vi "Initialize State.vi"(7 "dialog VI refnum":refnum<vi>, 8 "error in":errorcluster, 10 "VI refs":refnum<vi>[](array[refnum]), 11 "tree refnum":refnum<vi>) -> (0 "error out":errorcluster, 3 "state out":T1)   [LabVIEW 2010, in "NI_SE_Config Front Panel Layout.lvlib"]
uses:
  NI_SE_Config Front Panel Layout.lvlib
  State.ctl
  VI Info.ctl
  VI Panel Layout/VI Panel Layout.lvclass
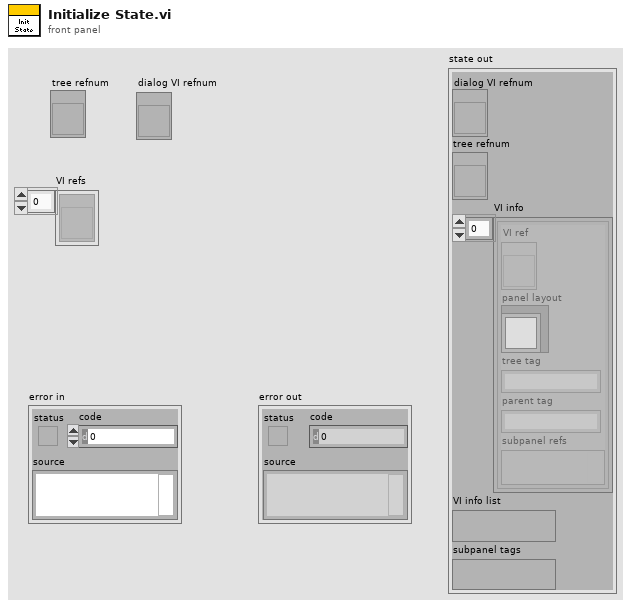
[diagram p1: front panel]
types:
  T1 = typedef "NI_SE_Config Front Panel Layout.lvlib/State.ctl" = cluster{"dialog VI refnum":refnum<vi>, "tree refnum":refnum<vi>, "VI info":T2[], "VI info list":variant, "subpanel tags":variant}
  T2 = typedef "NI_SE_Config Front Panel Layout.lvlib/VI Info.ctl" = cluster{"VI ref":refnum<vi>, "panel layout":refnum<class "VI Panel Layout.lvclass">, "tree tag":string, "parent tag":string, "subpanel refs":variant}
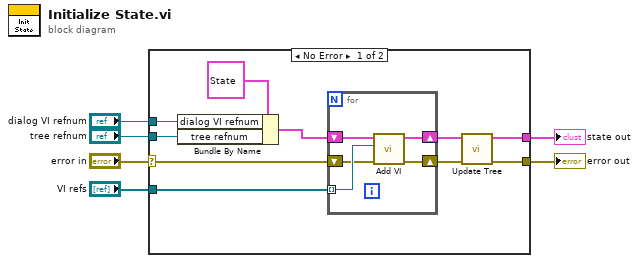
[diagram p0: block diagram]
diagram:
  n1 = case shown="No Error" "error in" {
    selector: "error in" -> [w14 w22]
    tunnel: [w11 w22] -> w5
    tunnel: [w13 _] -> w4
    tunnel: "tree refnum" -> [w7 _]
    tunnel: "VI refs" -> [w15 _]
    tunnel: "dialog VI refnum" -> [w8 _]
    frame No Error {
      n2 = Bundle By Name(cluster=T1 {"dialog VI refnum"=refnum, "tree refnum"=refnum, "VI info"=[], "VI info list"=variant, "subpanel tags"=variant} ("state out"), "dialog VI refnum"=w8, "tree refnum"=w7) -> (w9:T1)
      n3 = for {
        tunnel: w15 -> [w20] mode=indexing
        shift-right: [w17] -> w12
        shift-left: w14 -> [w18]
        shift-right: [w19] -> w10
        shift-left: w9 -> [w21]
        n4 = call "Add VI.vi"("error in"=w18, "VI ref"=w20, "state in"=w21) -> ("error out"=w17:errorcluster, "state out"=w19:T1)  [unwired: 7 in]
      }
      n5 = call "Update Tree.vi"("error in"=w12, "state in"=w10) -> ("error out"=w11:errorcluster, "state out"=w13:T1)  [unwired: 8 in]
    }
    frame Error {
    }
  }
  "state out" <- w4
  "error out" <- w5
